vi "Parse Auto Data.vi"(10 "Is Blue Alliance?":bool=TRUE, 11 "path":path) -> (1 "Zero Velocity?":bool[](array[boolean]), 2 "Velocities":T3[](array[typedef]), 3 "Positions":cluster{"x":dbl, "y":dbl, "th":dbl}[](array[cluster]), 5 "Commands out":cluster{"Time (s)":dbl, T1, bool}[](array[cluster]), 7 "Overall":cluster{"Time (s)":dbl, "Distance (ft)":dbl})   [LabVIEW 2020]
uses:
  swerve/Type Definitions/Data/Robot Velocities.ctl
  bordeaux-pathinator/Bordeaux/Types/Single Cmd Info.ctl
  <vilib>/picture/picture.llb/imagedata.ctl
  <vilib>/Analysis/coordinate.llb/2D Cartesian Coordinate Rotation (Scalar).vi
  <vilib>/Analysis/NI_AALPro.lvlib
panel:
  out "XY Graph":cluster{dbl[], dbl[]}[](graph)
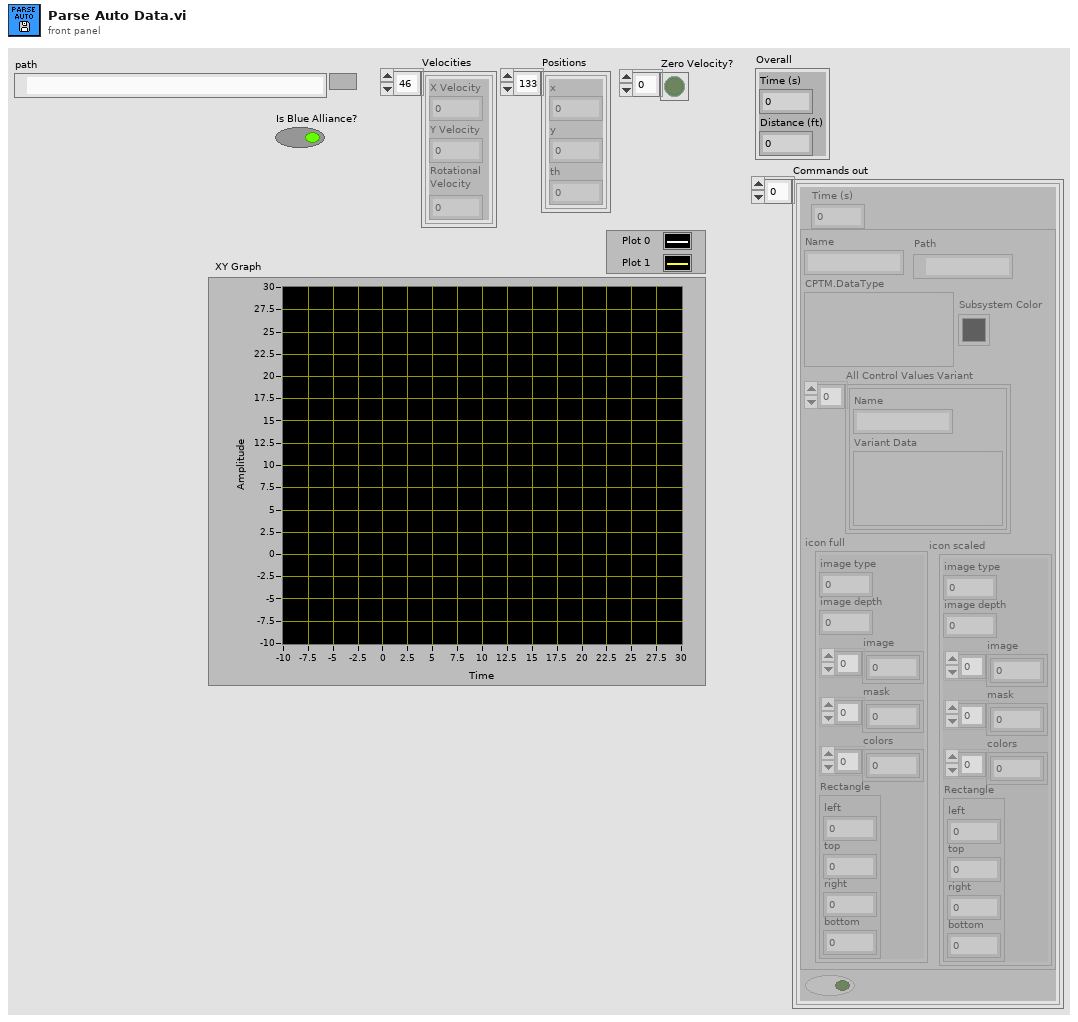
[diagram p1: front panel]
types:
  T1 = typedef "Single Cmd Info.ctl" = cluster{"Name":string, "CPTM.DataType":variant, "All Control Values Variant":cluster{"Name":string, "Variant Data":variant}[], "icon full":T2, "icon scaled":T2, "Path":path, "Subsystem Color":u32}
  T2 = typedef "imagedata.ctl" = cluster{"image type":i32, "image depth":i32, "image":u8[], "mask":u8[], "colors":u32[], "Rectangle":cluster{"left":i16, "top":i16, "right":i16, "bottom":i16}}
  T3 = typedef "Robot Velocities.ctl" = cluster{"X Velocity":dbl, "Y Velocity":dbl, "Rotational \nVelocity":dbl}
  T4 = typedef "Trajectory Data.ctl" = cluster{"Segment Name":string, "Type":T5, "Traj Pos Points":cluster{"x":dbl, "y":dbl, "th":dbl}[], "Traj Vel Points":cluster{"V":dbl, "Omega":dbl, "V vector":cluster{"y":dbl, "x":dbl}}[], "Accel Index":i32, "Decel Index":i32}[]
  T5 = typedef "Segment Type.ctl" = enum16{"Accel Straight", "Const Straight", "Blend", "Circle", "Bezier"}
  T6 = typedef "WPI_DriverStationAllianceInfo.ctl" = enum16{"Red", "Blue", "Invalid"}
  T7 = cluster{"V":dbl, "Omega":dbl, "V vector":cluster{"y":dbl, "x":dbl}}[]
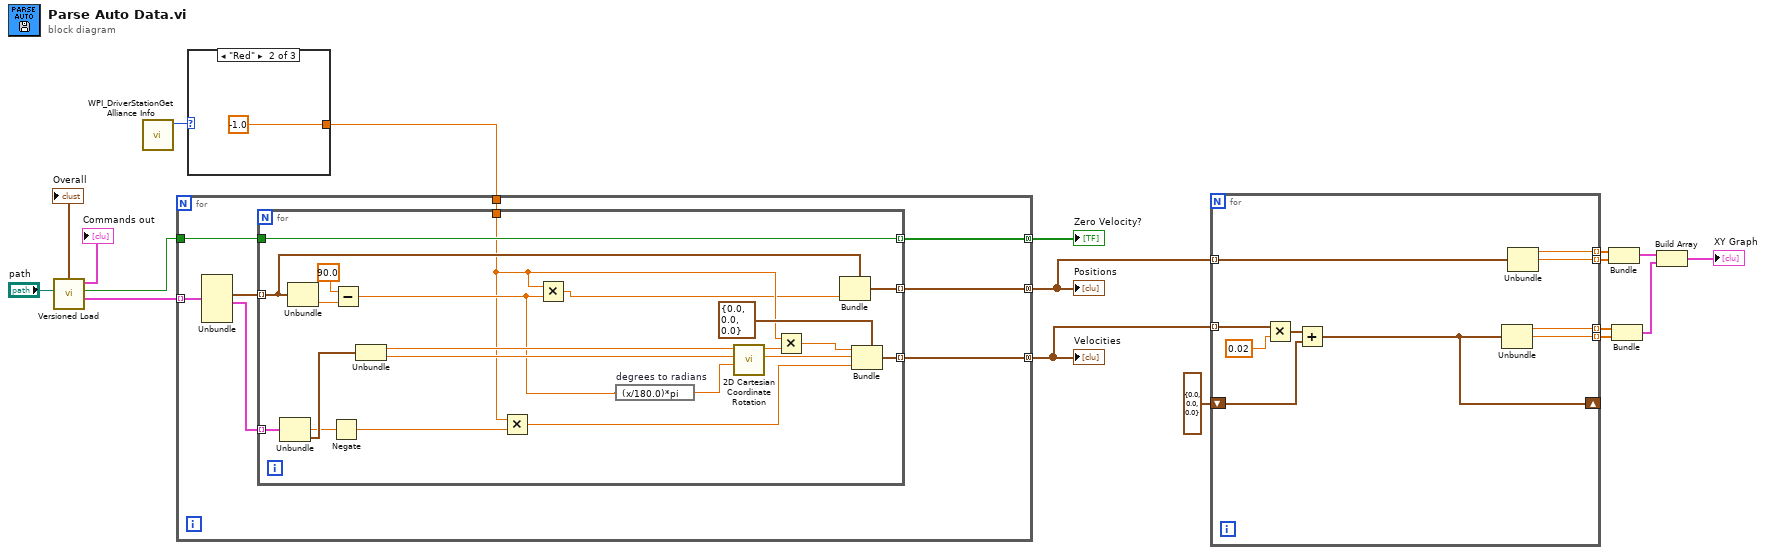
[diagram p0: block diagram]
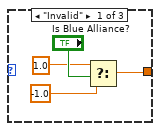
[diagram p2: hidden frame]
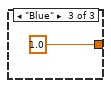
[diagram p3: hidden frame]
diagram:
  n1 = call "Versioned Load.vi"("path"="path") -> ("Trajectory Data"=w17:T4, "Zero V"=w14:bool, "Commands out"=→"Commands out":cluster{"Time (s)":dbl, T1, bool}[], "Overall"=→"Overall":cluster{"Time (s)":dbl, "Distance (ft)":dbl})  [unwired: 3 in, 4 out]
  n2 = call <vilib>:"WPI_DriverStationGet Alliance Info.vi"() -> ("Alliance"=w16:T6)  [unwired: 6 in, 5 out]
  n3 = case shown="\"Red\"" w16 {
    tunnel: [w19 -1.0 1.0] -> w15
    frame "Invalid" {
      n4 = Select(t=1.0, s="Is Blue Alliance?", f=-1.0) -> (s? t:f=w19:dbl)
    }
    frame "Red" {
    }
    frame "Blue" {
    }
  }
  n5 = for {
    tunnel: w17 -> [w32] mode=indexing
    tunnel: [w29] -> w10 mode=concatenating
    tunnel: w15 -> [w28]
    tunnel: [w25] -> w9 mode=concatenating
    tunnel: w14 -> [w27]
    tunnel: [w26] -> w13 mode=concatenating
    n6 = Unbundle(w32) -> ("Traj Pos Points"=w31:cluster{"x":dbl, "y":dbl, "th":dbl}[], "Traj Vel Points"=w30:T7)  [unwired: 4 out]
    n7 = for {
      tunnel: w31 -> [w51] mode=indexing
      tunnel: w30 -> [w49] mode=indexing
      tunnel: [w50] -> w29 mode=indexing
      tunnel: w28 -> [w34]
      tunnel: [w41] -> w25 mode=indexing
      tunnel: w27 -> [w38]
      tunnel: [w38] -> w26 mode=indexing
      n8 = Unbundle(w49) -> ("Omega"=w37:dbl, "V vector"=w48:cluster{"y":dbl, "x":dbl})  [unwired: 1 out]
      n9 = Unbundle(w51) -> ("th"=w53:dbl)  [unwired: 2 out]
      n10 = Negate(x=w37) -> (-x=w36:dbl)
      n11 = Subtract(x=90.0, y=w53) -> (x-y=w35:dbl)
      n12 = Unbundle(w48) -> ("y"=w46:dbl, "x"=w45:dbl)
      n13 = Multiply(x=w34, y=w36) -> (x*y=w43:dbl)
      n14 = Multiply(x=w34, y=w35) -> (x*y=w33:dbl)
      n15 = expression code="(x/180.0)*pi" "degrees to radians"(w35) -> (w47:dbl)
      n16 = call-poly <vilib>:"2D Cartesian Coordinate Rotation.vi"("theta"=w47, "y"=w45, "x"=w46) -> ("y out"=w44:dbl, "x out"=w40:dbl)  [unwired: 6 in, 1 out]
      n17 = Multiply(x=w34, y=w40) -> (x*y=w39:dbl)
      n18 = Bundle(cluster=w51, "th"=w33) -> (w50:cluster{"x":dbl, "y":dbl, "th":dbl})  [unwired: 2 in]
      n19 = Bundle(cluster=T3 {"X Velocity"=0.0, "Y Velocity"=0.0, "Rotational \nVelocity"=0.0} ("Robot Velocities"), "X Velocity"=w39, "Y Velocity"=w44, "Rotational \nVelocity"=w43) -> (w41:T3)
    }
  }
  "Positions" <- w10
  "Velocities" <- w9
  "Zero Velocity?" <- w13
  n20 = for {
    tunnel: w10 -> [w63] mode=indexing
    tunnel: w9 -> [w60] mode=indexing
    tunnel: [w62] -> w8 mode=indexing
    tunnel: [w61] -> w7 mode=indexing
    shift-right: [w56] -> _
    shift-left: T3 {"X Velocity"=0.0, "Y Velocity"=0.0, "Rotational \nVelocity"=0.0} ("Robot Velocities") -> [w57]
    tunnel: [w55] -> w5 mode=indexing
    tunnel: [w54] -> w4 mode=indexing
    n21 = Multiply(x=w60, y=0.02) -> (x*y=w58:T3)
    n22 = Add(x=w58, y=w57) -> (x+y=w56:T3)
    n23 = Unbundle(w56) -> ("X Velocity"=w55:dbl, "Y Velocity"=w54:dbl)  [unwired: 1 out]
    n24 = Unbundle(w63) -> ("x"=w62:dbl, "y"=w61:dbl)  [unwired: 1 out]
  }
  n25 = Bundle(w8, w7) -> (w3:cluster{dbl[], dbl[]})  [unwired: 1 in]
  n26 = Bundle(w5, w4) -> (w2:cluster{dbl[], dbl[]})  [unwired: 1 in]
  n27 = Build Array(w3, w2) -> (→"XY Graph":cluster{dbl[], dbl[]}[])
